vi "Transform to Plain Job and Machine Gaps Array.vi"(8 "v":i32, 9 "Job Gaps":T1[][](array[typedef]), 10 "u":i32, 11 "Machine Gaps":T1[][](array[typedef])) -> (1 "Job Gaps Array":i32[][](array[numeric]), 3 "Machine Gaps Array":i32[][](array[numeric]))   [LabVIEW 2013, in "Scheduler.lvclass"]
uses:
  Scheduler.lvclass
  Controls/GapStructure4FIFOEngine.ctl
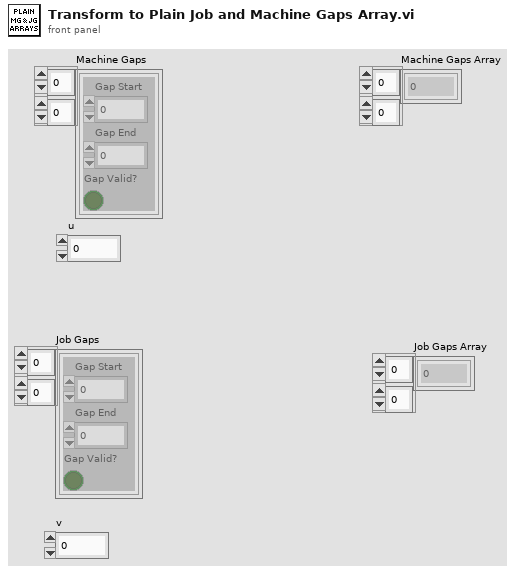
[diagram p1: front panel]
types:
  T1 = typedef "Scheduler.lvclass/GapStructure4FIFOEngine.ctl" = cluster{"Gap Start":i32, "Gap End":i32, "Gap Valid?":bool}
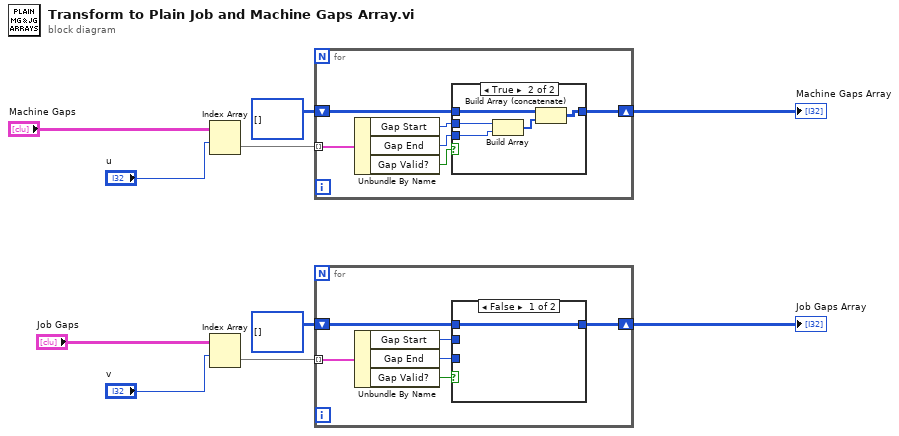
[diagram p0: block diagram]
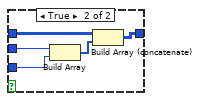
[diagram p2: hidden frame]
diagram:
  n1 = Index Array(array="Machine Gaps", index (row)="u") -> (element=w4:T1[])  [unwired: 1 in]
  n2 = Index Array(array="Job Gaps", index (row)="v") -> (element=w3:T1[])  [unwired: 1 in]
  n3 = for {
    tunnel: w4 -> [w16] mode=indexing
    shift-right: [w14] -> w6
    shift-left: i32[][] [] -> [w15]
    n4 = Unbundle By Name(w16) -> ("Gap Start"=w12:i32, "Gap End"=w11:i32, "Gap Valid?"=w13:bool)
    n5 = case shown="True" w13 {
      tunnel: w12 -> [_ w22]
      tunnel: w11 -> [_ w21]
      tunnel: w15 -> [w17 w19]
      tunnel: [w17 w18] -> w14
      frame False {
      }
      frame True {
        n6 = Build Array(w22, w21) -> (w20:i32[])
        n7 = Build Array (concatenate)(w19, w20) -> (w18:i32[][])
      }
    }
  }
  "Machine Gaps Array" <- w6
  n8 = for {
    tunnel: w3 -> [w28] mode=indexing
    shift-right: [w24] -> w5
    shift-left: i32[][] [] -> [w25]
    n9 = Unbundle By Name(w28) -> ("Gap Start"=w27:i32, "Gap End"=w26:i32, "Gap Valid?"=w23:bool)
    n10 = case shown="False" w23 {
      tunnel: w27 -> [_ w34]
      tunnel: w26 -> [_ w33]
      tunnel: w25 -> [w29 w31]
      tunnel: [w29 w30] -> w24
      frame False {
      }
      frame True {
        n11 = Build Array(w34, w33) -> (w32:i32[])
        n12 = Build Array (concatenate)(w31, w32) -> (w30:i32[][])
      }
    }
  }
  "Job Gaps Array" <- w5
